vi "DmmPwr Simulator Acquire Single.vi"() -> ()   [LabVIEW 2013]
doc: "This example shows how to configure a measurement and take a reading."
uses:
  <instrlib>/DmmPwr Simulator/DmmPwr Simulator.lvlib
panel:
  in  "Power Supple Output Level":dbl=7.2 format="%#_13g"
  in  "Function (0: DC Volts)":u16(ring) items=["DC Volts", "AC Volts", "DC Current", "AC Current"]
  in  "Auto Range":bool=TRUE
  in  "Manual Range":dbl=1.0
  out "Measurement":dbl
  in  "VISA resource name":refnum<visa-resource-name>="TCPIP::localhost::9997::SOCKET"
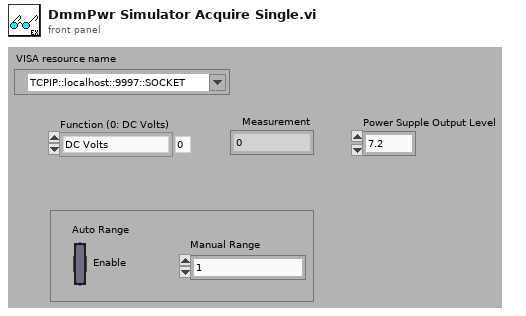
[diagram p1: front panel]
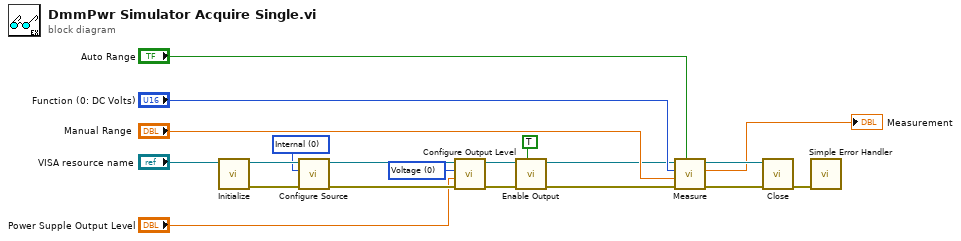
[diagram p0: block diagram]
diagram:
  w3 = u16 0 items=["Voltage", "Current"] ("Output Type (0: Voltage)")
  w10 = u16 0 items=["Internal", "External"] ("Source (Internal)")
  n1 = call <instrlib>:"Initialize.vi"("VISA resource name"="VISA resource name") -> ("error out"=w11:errorcluster, "VISA resource name out"=w12:refnum<visa-resource-name>)  [unwired: 9 in]
  n2 = call <instrlib>:"Configure Source.vi"("error in (no error)"=w11, "Source (Internal)"=w10, "VISA resource name"=w12) -> ("error out"=w7:errorcluster, "VISA resource name out"=w9:refnum<visa-resource-name>)  [unwired: 7 in]
  n3 = call <instrlib>:"Configure Output Level.vi"("error in (no error)"=w7, "Output Level (0)"="Power Supple Output Level", "Output Type (0: Voltage)"=w3, "VISA resource name"=w9) -> ("error out"=w6:errorcluster, "VISA resource name out"=w8:refnum<visa-resource-name>)  [unwired: 6 in]
  n4 = call <instrlib>:"Enable Output.vi"("Enable Output (F: Disable)"=TRUE, "error in (no error)"=w6, "VISA resource name"=w8) -> ("error out"=w5:errorcluster, "VISA resource name out"=w4:refnum<visa-resource-name>)  [unwired: 7 in]
  n5 = call <instrlib>:"Measure.vi"("Auto Range (T:Enable)"="Auto Range", "error in"=w5, "Manual Range (1.0)"="Manual Range", "Function (0: DC Volts)"="Function (0: DC Volts)", "VISA resource name"=w4) -> ("error out"=w14:errorcluster, "Measured Value"=→"Measurement":dbl, "VISA resource name out"=w18:refnum<visa-resource-name>)  [unwired: 4 in]
  n6 = call <instrlib>:"Close.vi"("error in (no error)"=w14, "VISA resource name"=w18) -> ("error out"=w20:errorcluster)  [unwired: 9 in]
  n7 = call <vilib>:"Simple Error Handler.vi"("error in (no error)"=w20) -> ()  [unwired: 4 in, 5 out]
